vi "Actual Sample Rate Core.vi"(8 "error in (no error)":errorcluster, 11 "IVI_Scope in":refnum<class "IVI_Scope.lvclass">) -> (0 "error out":errorcluster, 2 "sample rate":dbl[unit] caption="sample rate (samples/s)" format="%^.2e", 3 "IVI_Scope out":refnum<class "IVI_Scope.lvclass">)   [LabVIEW 2013, in "IVI_Scope.lvlib" / "IVI_Scope.lvclass"]
doc: "This VI returns the effective sample rate of the acquired waveform using the current configuration in samples per second."
uses:
  IVI_Scope.lvclass
  IVI_Scope.lvclass/IVI_Scope.ctl
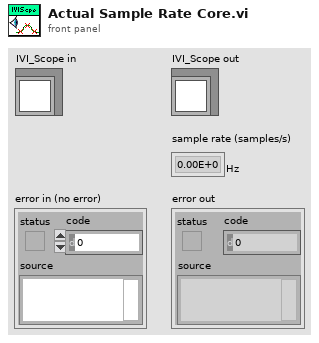
[diagram p1: front panel]
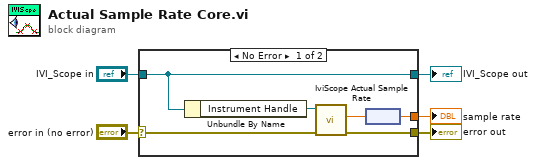
[diagram p0: block diagram]
diagram:
  n1 = case shown="No Error" "error in (no error)" {
    selector: "error in (no error)" -> [w9 w13]
    tunnel: [w8 w13] -> w4
    tunnel: [w11 w12] -> w2
    tunnel: "IVI_Scope in" -> [w11 w12]
    tunnel: [w6 _] -> w1
    frame No Error {
      n2 = Unbundle By Name(w11) -> ("Instrument Handle"=w10:refnum<k15>)
      n3 = call <vilib>:"IviScope Actual Sample Rate.vi"("error in (no error)"=w9, "instrument handle"=w10) -> ("error out"=w8:errorcluster, "sample rate"=w7:dbl)  [unwired: 7 in, 1 out]
      n4 = node(w7) -> (w6:dbl[unit])
    }
    frame Error {
    }
  }
  "error out" <- w4
  "IVI_Scope out" <- w2
  "sample rate" <- w1
